vi "下拉列表-按值查找项名.vi"(2 "error in (no error)":errorcluster caption="错误输入（无错误）", 3 "下拉列表":refnum<vi>) -> (0 "error out":errorcluster caption="错误输出", 1 "项名":string)   [LabVIEW 2014]
doc: "该模板用于创建子VI。"
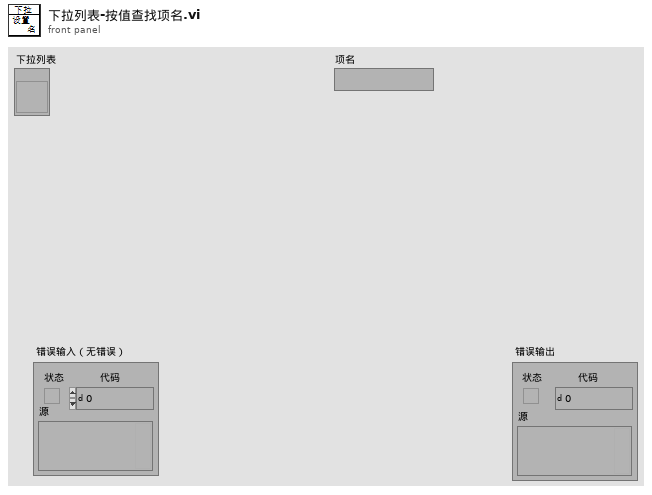
[diagram p1: front panel]
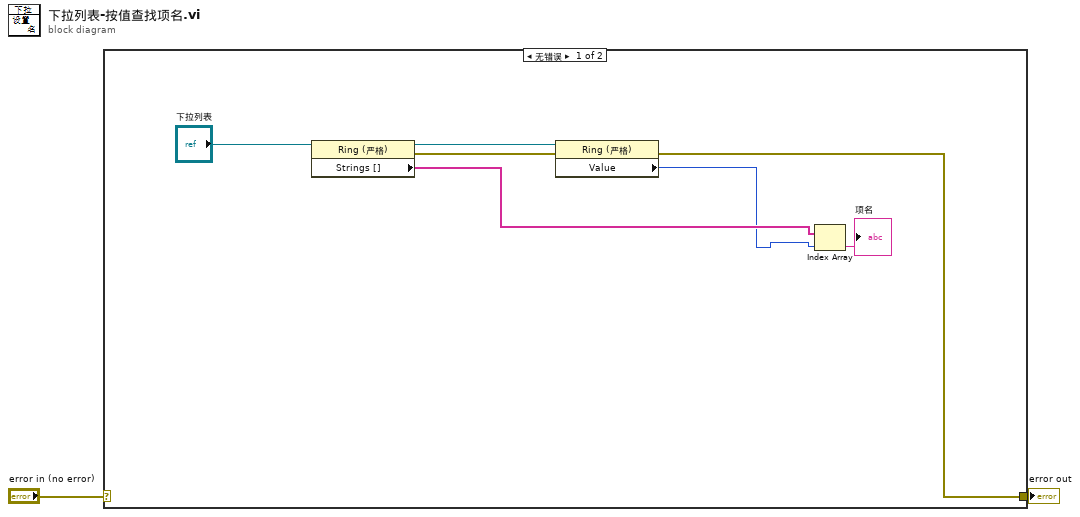
[diagram p0: block diagram]
diagram:
  n1 = case shown="无错误" "error in (no error)" {
    selector: "error in (no error)" -> [_ w10]
    tunnel: [w6 w10] -> w1
    frame No Error {
      n2 = property class="Ring (严格)"(reference="下拉列表") -> (reference out=w8:refnum<vi>, error out=w7:errorcluster, "Strings []"=w5:string[])  [unwired: 1 in]
      n3 = property class="Ring (严格)"(reference=w8, error in=w7) -> (error out=w6:errorcluster, "Value"=w4:u16)  [unwired: 1 out]
      n4 = Index Array(array=w5, index=w4) -> (element=→"项名":string)
    }
    frame Error {
    }
  }
  "error out" <- w1
